vi "sensor check.vi"(8 "error in":errorcluster, 10 "input cluster":T1, 11 "Gantry In":refnum<k24>) -> (0 "error out":errorcluster, 1 "Wrong Orientation?":bool, 2 "output cluster":T1, 3 "Gantry Out":refnum<k24>)   [LabVIEW 2021, in "Component Tray.lvclass"]
uses:
  Component Tray.lvclass
  Controller/Motion/A3200/A3200.lvclass
  Controller/Camera/Machine Vision.ctl
  Controller/Camera/Camera.lvclass
  Find Component.ctl
  C:/Program Files (x86)/Aerotech/A3200/LabVIEW/2010/Bin/Aerotech.A3200.dll
  Program Files (x86)/Aerotech/A3200/LabVIEW/2010/Bin/Aerotech.A3200.dll
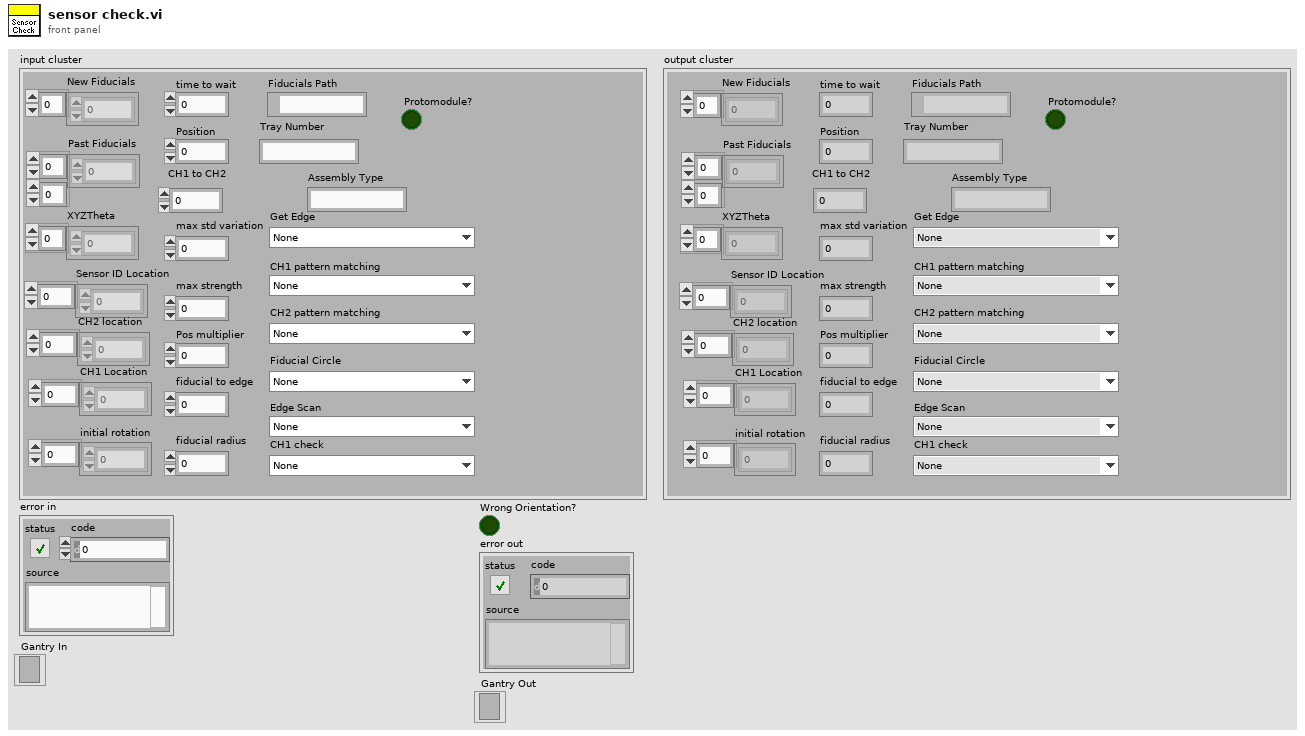
[diagram p1: front panel]
types:
  T1 = typedef "Component Tray.lvclass/Find Component.ctl" = cluster{"New Fiducials":dbl[], "Past Fiducials":dbl[][], "XYZTheta":dbl[], "Fiducials Path":path, "Position":i32, "CH1 Location":dbl[], "Sensor ID Location":dbl[], "initial rotation":dbl[], "CH2 location":dbl[], "max std variation":dbl, "max strength":dbl, "CH2 pattern matching":T2, "Fiducial Circle":T2, "Get Edge":T2, "Pos multiplier":dbl, "time to wait":u32, "fiducial to edge":dbl, "Protomodule?":bool, "Assembly Type":string, "CH1 to CH2":dbl, "Tray Number":string, "fiducial radius":dbl, "4 fiducials?":bool, "CH1 check":T2, "Edge Scan":T2, "CH1 pattern matching":T2, "Sensor Thickness":dbl}
  T2 = typedef "Camera.lvclass/Machine Vision.ctl" = enum16{"None", "Assembly Tray Circle", "Assembly Tray Fiducial", "Partial Hexaboard", "sensor edge init", "HB edge init", "sensor edge pos1", "sensor edge pos2", "HB edge pos1", "HB edge pos2", "Sensor CH1-2", "HB CH1", "HB CH2", "V3 Sensor Circle", "Hexaboard Circle", "sensor CH1 check", "HB CH1 check "}
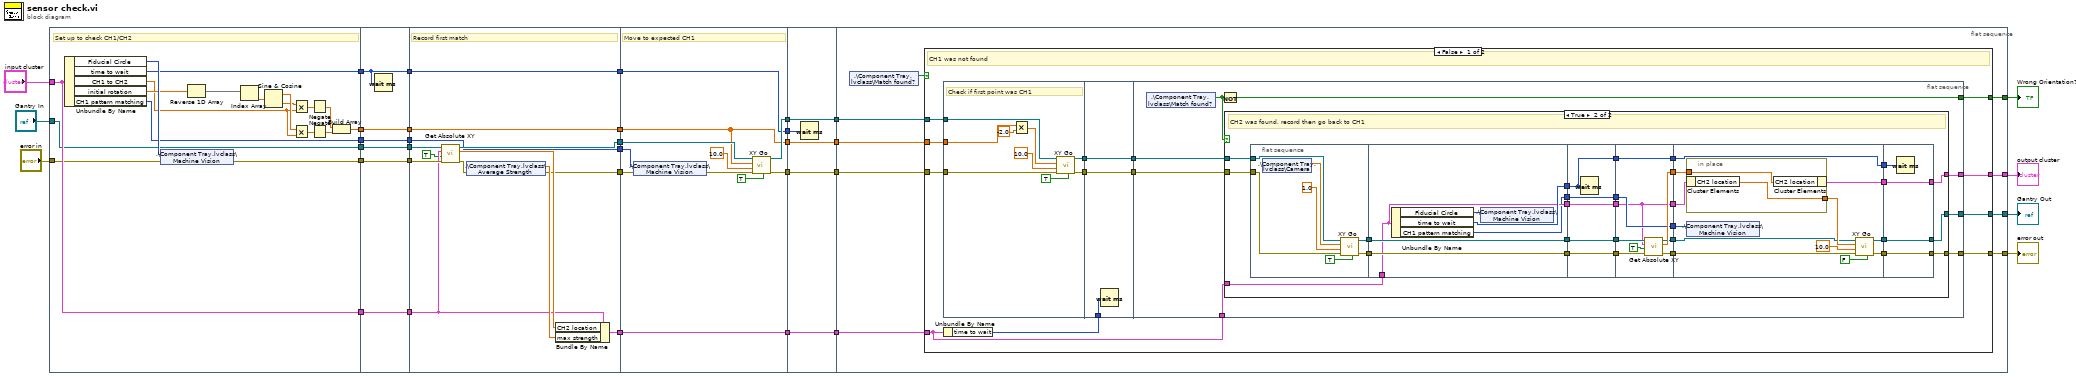
[diagram p0: block diagram]
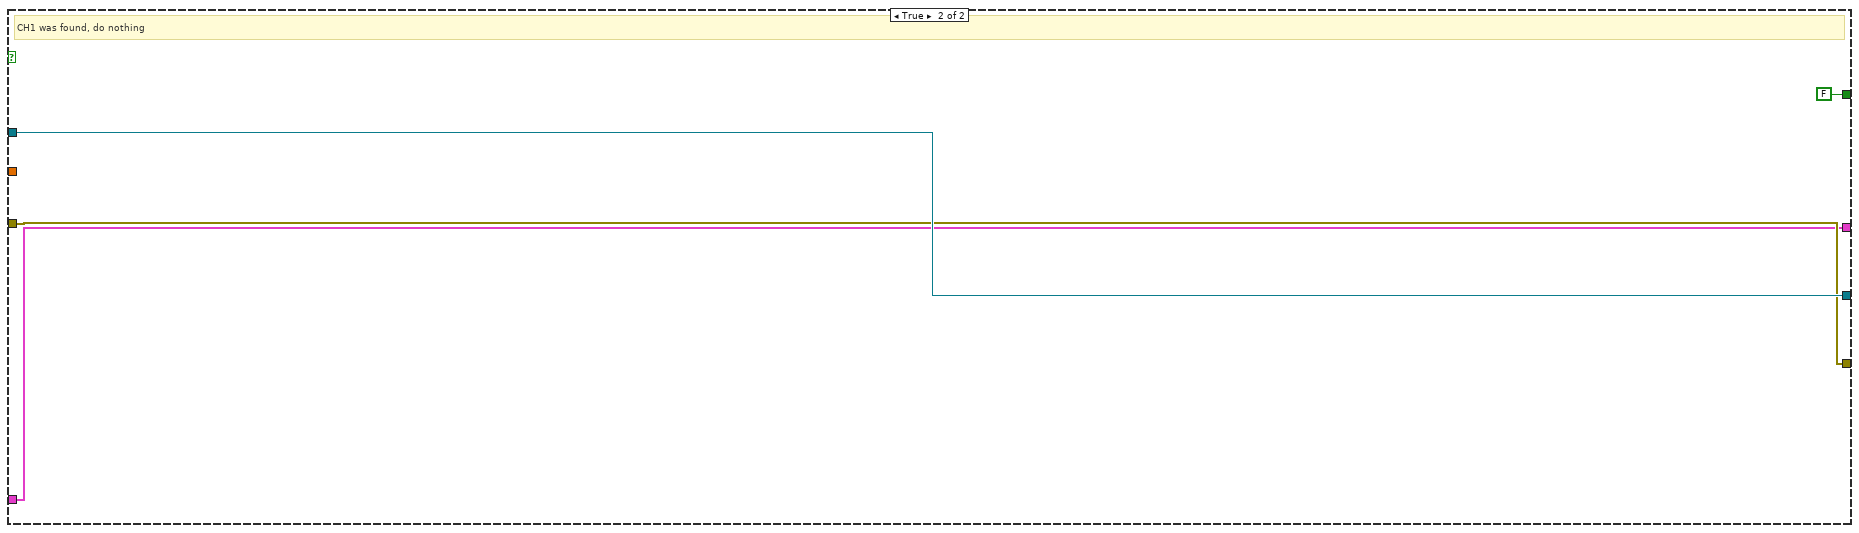
[diagram p3: hidden frame]
diagram:
  n1 = flat-sequence {
    tunnel: [w41] -> w21
    tunnel: [w39] -> w19
    tunnel: [w42] -> w17
    tunnel: [w51] -> w15
    tunnel: [w44] -> w13
    tunnel: [w43] -> w11
    tunnel: "input cluster" -> [w42]
    tunnel: "error in" -> [w40]
    tunnel: "Gantry In" -> [w41]
    tunnel: w21 -> [w58]
    tunnel: [w58] -> w20
    tunnel: w19 -> [w57]
    tunnel: [w57] -> w18
    tunnel: w17 -> [w56]
    tunnel: [w56] -> w16
    tunnel: w15 -> [w55]
    tunnel: [w55] -> w14
    tunnel: w13 -> [w54]
    tunnel: [w54] -> w12
    tunnel: w11 -> [w53]
    tunnel: [w53] -> w10
    tunnel: w20 -> [w70]
    tunnel: w18 -> [w69]
    tunnel: w16 -> [w60]
    tunnel: w14 -> [w64]
    tunnel: w12 -> [w67]
    tunnel: [w68] -> w34
    tunnel: [w61] -> w33
    tunnel: [w67] -> w32
    tunnel: [w66] -> w31
    tunnel: [w65] -> w30
    tunnel: w10 -> [w65]
    tunnel: [w64] -> w29
    tunnel: w34 -> [w82]
    tunnel: w33 -> [w73]
    tunnel: w32 -> [w74]
    tunnel: w31 -> [w79]
    tunnel: w30 -> [w76]
    tunnel: [w77] -> w9
    tunnel: [w78] -> w7
    tunnel: [w82] -> w5
    tunnel: w29 -> [w75]
    tunnel: [w75] -> w3
    tunnel: [w74] -> w2
    tunnel: w9 -> [w87]
    tunnel: [w87] -> w8
    tunnel: w7 -> [w86]
    tunnel: [w86] -> w6
    tunnel: w5 -> [w85]
    tunnel: [w85] -> w4
    tunnel: w3 -> [w84]
    tunnel: w2 -> [w83]
    tunnel: [w83] -> w1
    tunnel: [w89] -> w24
    tunnel: [w92] -> w23
    tunnel: [w94] -> w22
    tunnel: w8 -> [w95]
    tunnel: w6 -> [w93]
    tunnel: w4 -> [w90]
    tunnel: w1 -> [w91]
    tunnel: [w88] -> w25
    frame #0 {
      # "Set up to check CH1/CH2"
      n2 = Unbundle By Name(w42) -> ("Fiducial Circle"=w52:T2, "time to wait"=w51:u32, "CH1 to CH2"=w45:dbl, "initial rotation"=w46:dbl[], "CH1 pattern matching"=w43:T2)
      n3 = shared-variable ".\\Component Tray.lvclass\\Machine Vision"(w52, error in=w40) -> (error out=w39:errorcluster)
      n4 = Reverse 1D Array(array=w46) -> (reversed array=w47:dbl[])
      n5 = Index Array(array=w47) -> (element=w50:dbl)  [unwired: 1 in]
      n6 = Sine & Cosine(0:w50) -> (1:w49:dbl, 2:w48:dbl)
      n7 = Multiply(x=w48, y=w45) -> (x*y=w36:dbl)
      n8 = Multiply(x=w49, y=w45) -> (x*y=w38:dbl)
      n9 = Negate(x=w36) -> (-x=w35:dbl)
      n10 = Negate(x=w38) -> (-x=w37:dbl)
      n11 = Build Array(w35, w37) -> (w44:dbl[])
    }
    frame #1 {
      n12 = Wait (ms)(milliseconds to wait=w55) -> ()  [unwired: 1 out]
    }
    frame #2 {
      # "Record first match"
      n13 = call "Get Absolute XY.vi"("error in (no error)"=w69, 9:TRUE ("Fiducial?"), "input cluster"=w60, "Gantry In"=w70) -> ("error out"=w62:errorcluster, "Abs XY"=w71:dbl[], "Gantry Out"=w66:refnum<k24>)  [unwired: 5 in]
      n14 = shared-variable ".\\Component Tray.lvclass\\Average Strength"(error in=w62) -> (w63:dbl, error out=w61:errorcluster)
      n15 = Bundle By Name(cluster=w60, "CH2 location"=w71, "max strength"=w63) -> (w68:T1)
    }
    frame #3 {
      # "Move to expected CH1"
      n16 = shared-variable ".\\Component Tray.lvclass\\Machine Vision"(w76, error in=w73) -> (error out=w72:errorcluster)
      n17 = call "XY Go.vi"("Increment?"=TRUE, "error in (no error)"=w72, "Speed"=10.0, "XY In"=w74, "Gantry In"=w79) -> ("error out"=w78:errorcluster, "Gantry Out"=w77:refnum<k24>)  [unwired: 4 in, 1 out]
    }
    frame #4 {
      n18 = Wait (ms)(milliseconds to wait=w84) -> ()  [unwired: 1 out]
    }
    frame #5 {
      n19 = shared-variable ".\\Component Tray.lvclass\\Match found?"() -> (w96:bool)  [unwired: 1 in, 1 out]
      n20 = case shown="False" w96 {
        tunnel: w95 -> [w109 w209]
        tunnel: [w108 w209] -> w94
        tunnel: w93 -> [w107 w208]
        tunnel: [w106 w208] -> w92
        tunnel: w91 -> [w105 _]
        tunnel: w90 -> [w104 w207]
        tunnel: [w102 w207] -> w89
        tunnel: [w103 FALSE] -> w88
        frame False {
          # "CH1 was not found"
          n21 = flat-sequence {
            tunnel: w109 -> [w118]
            tunnel: w107 -> [w115]
            tunnel: w105 -> [w112]
            tunnel: [w117] -> w101
            tunnel: [w114] -> w99
            tunnel: w101 -> [w121]
            tunnel: [w121] -> w100
            tunnel: w99 -> [w120]
            tunnel: [w120] -> w98
            tunnel: w97 -> [w119]
            tunnel: [w124] -> w106
            tunnel: [w126] -> w108
            tunnel: w100 -> [w127]
            tunnel: w98 -> [w125]
            tunnel: [w128] -> w103
            tunnel: w104 -> [w123]
            tunnel: [w122] -> w102
            frame #0 {
              # "Check if first point was CH1"
              n22 = Multiply(x=w112, y=-2.0) -> (x*y=w111:dbl[])
              n23 = call "XY Go.vi"("Increment?"=TRUE, "error in (no error)"=w115, "Speed"=10.0, "XY In"=w111, "Gantry In"=w118) -> ("error out"=w114:errorcluster, "Gantry Out"=w117:refnum<k24>)  [unwired: 4 in, 1 out]
            }
            frame #1 {
              n24 = Wait (ms)(milliseconds to wait=w119) -> ()  [unwired: 1 out]
            }
            frame #2 {
              n25 = shared-variable ".\\Component Tray.lvclass\\Match found?"() -> (w129:bool)  [unwired: 1 in, 1 out]
              n26 = Not(x=w129) -> (.not. x?=w128:bool)
              n27 = case shown="True" w129 {
                tunnel: w127 -> [w132 w160]
                tunnel: [w132 w159] -> w126
                tunnel: w125 -> [w130 w158]
                tunnel: [w130 w155] -> w124
                tunnel: w123 -> [w131 w156]
                tunnel: [w131 w153] -> w122
                frame False {
                  # "Only one fiducial was found, throw an error"
                }
                frame True {
                  # "CH2 was found, record then go back to CH1"
                  n28 = flat-sequence {
                    tunnel: w160 -> [w167]
                    tunnel: w158 -> [w165]
                    tunnel: [w166] -> w157
                    tunnel: [w161] -> w154
                    tunnel: w157 -> [w173]
                    tunnel: w156 -> [w169]
                    tunnel: [w173] -> w142
                    tunnel: [w171] -> w140
                    tunnel: w154 -> [w170]
                    tunnel: [w170] -> w138
                    tunnel: [w169] -> w136
                    tunnel: [w168] -> w134
                    tunnel: w142 -> [w178]
                    tunnel: [w178] -> w141
                    tunnel: w140 -> [w177]
                    tunnel: [w177] -> w139
                    tunnel: w138 -> [w176]
                    tunnel: [w176] -> w137
                    tunnel: w136 -> [w175]
                    tunnel: [w175] -> w135
                    tunnel: w134 -> [w174]
                    tunnel: [w174] -> w133
                    tunnel: w141 -> [w187]
                    tunnel: w139 -> [w182]
                    tunnel: w137 -> [w186]
                    tunnel: w135 -> [w180]
                    tunnel: [w180] -> w148
                    tunnel: [w185] -> w147
                    tunnel: [w184] -> w146
                    tunnel: [w183] -> w145
                    tunnel: [w182] -> w144
                    tunnel: [w181] -> w143
                    tunnel: w133 -> [w181]
                    tunnel: [w189] -> w152
                    tunnel: [w190] -> w151
                    tunnel: [w191] -> w150
                    tunnel: [w199] -> w149
                    tunnel: w148 -> [w197]
                    tunnel: w147 -> [w196]
                    tunnel: w146 -> [w194]
                    tunnel: w145 -> [w192]
                    tunnel: w144 -> [w199]
                    tunnel: w143 -> [w188]
                    tunnel: [w203] -> w153
                    tunnel: [w204] -> w155
                    tunnel: [w205] -> w159
                    tunnel: w152 -> [w205]
                    tunnel: w151 -> [w204]
                    tunnel: w150 -> [w203]
                    tunnel: w149 -> [w202]
                    frame #0 {
                      n29 = shared-variable ".\\Component Tray.lvclass\\Camera"() -> (w164:dbl[])  [unwired: 1 in, 1 out]
                      n30 = call "XY Go.vi"("Increment?"=TRUE, "error in (no error)"=w165, "Speed"=1.0, "XY In"=w164, "Gantry In"=w167) -> ("error out"=w161:errorcluster, "Gantry Out"=w166:refnum<k24>)  [unwired: 4 in, 1 out]
                    }
                    frame #1 {
                      n31 = Unbundle By Name(w169) -> ("Fiducial Circle"=w172:T2, "time to wait"=w171:u32, "CH1 pattern matching"=w168:T2)
                      n32 = shared-variable ".\\Component Tray.lvclass\\Machine Vision"(w172) -> ()  [unwired: 1 in, 1 out]
                    }
                    frame #2 {
                      n33 = Wait (ms)(milliseconds to wait=w177) -> ()  [unwired: 1 out]
                    }
                    frame #3 {
                      n34 = call "Get Absolute XY.vi"("error in (no error)"=w186, 9:TRUE ("Fiducial?"), "input cluster"=w180, "Gantry In"=w187) -> ("error out"=w184:errorcluster, "Abs XY"=w185:dbl[], "Gantry Out"=w183:refnum<k24>)  [unwired: 5 in]
                    }
                    frame #4 {
                      n35 = in-place {
                        in-place-border: w196 -> [w201]
                        in-place-border: [w200] -> w198
                        n36 = in-place-cluster #1(w197) -> ("CH2 location"=w200:dbl[])
                        n37 = in-place-cluster #1("CH2 location"=w201) -> (w191:T1)
                      }
                      n38 = shared-variable ".\\Component Tray.lvclass\\Machine Vision"(w188) -> ()  [unwired: 1 in, 1 out]
                      n39 = call "XY Go.vi"("Increment?"=FALSE, "error in (no error)"=w194, "Speed"=10.0, "XY In"=w198, "Gantry In"=w192) -> ("error out"=w190:errorcluster, "Gantry Out"=w189:refnum<k24>)  [unwired: 4 in, 1 out]
                    }
                    frame #5 {
                      n40 = Wait (ms)(milliseconds to wait=w202) -> ()  [unwired: 1 out]
                    }
                  }
                }
              }
            }
          }
          n41 = Unbundle By Name(w104) -> ("time to wait"=w97:u32)
        }
        frame True {
          # "CH1 was found, do nothing"
        }
      }
    }
  }
  "Wrong Orientation?" <- w25
  "output cluster" <- w24
  "error out" <- w23
  "Gantry Out" <- w22
